vi "ForLoopArray.vi"() -> ()   [LabVIEW 2019]
panel:
  in  "Array 2":dbl[](array[numeric])
  out "element 2":dbl
  out "element":dbl
  in  "Array":dbl[](array[numeric])
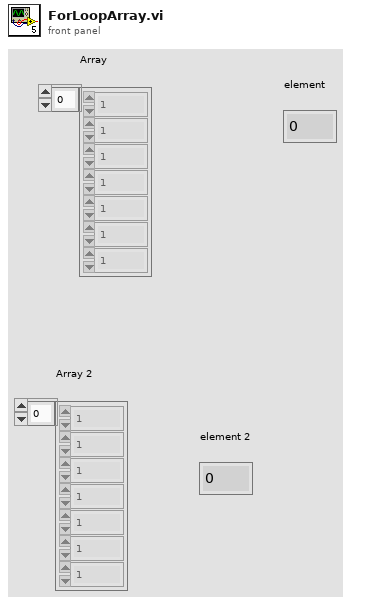
[diagram p1: front panel]
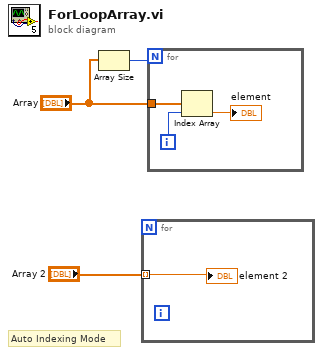
[diagram p0: block diagram]
diagram:
  # "Auto Indexing Mode"
  n1 = Array Size(array="Array") -> (size(s)=w3:i32)
  n2 = for {
    tunnel: "Array 2" -> [w4] mode=indexing
    "element 2" <- w4
  }
  n3 = for {
    N: w3 -> [_]
    tunnel: "Array" -> [w7]
    i -> [w6]
    n4 = Index Array(array=w7, index=w6) -> (element=→"element":dbl)
  }
